vi "Chemical_Plant.vi"() -> ()   [LabVIEW 2024]
uses:
  <vilib>/addons/control/pid/pid.llb/PID (DBL).vi
  <vilib>/addons/control/pid/NI_PID_pid.lvlib
panel:
  in  "CHEMICAL PLANT":enum32{"MAIN_PANEL", "DSC", "FUNCTIONAL"}(tab)
  out "TRANS":bool
  in  "TRANSFORMER":bool
  out "Boolean 18":bool
  out "IL":dbl(knob) scale=0.0..200.0
  out "UL":dbl(knob) scale=0.0..10000.0
  out "TEMP 2":dbl(slide)=35.0 scale=0.0..1000.0
  in  "Power 2":i64(knob)=10 scale=0.0..10.0
  in  "Setpoint °C 2":dbl(knob)=1000.0 min=0.0 max=1000.0 step=1.0 scale=0.0..1000.0
  in  "CONV":bool
  out "Boolean 17":bool
  out "ATM":dbl(knob) scale=0.0..10.0
  out "Boolean 16":bool
  out "Boolean 15":bool
  in  "AV":bool
  in  "AP":bool
  out "Boolean 14":bool
  out "Boolean 13":bool
  in  "MV":bool
  in  "MP":bool
  out "Boolean 12":bool
  out "Boolean 11":bool
  in  "WV":bool
  in  "WP":bool
  out "Boolean 10":bool
  in  "CCV 2":bool
  out "Boolean 9":bool
  out "Boolean 8":bool
  in  "CCV":bool
  in  "CCP":bool
  in  "Set  limit":dbl=4.5 min=0.0 max=10.0 step=0.5 format="%#_2g"
  in  "COMP":bool
  out "Boolean 5":bool
  out "I_opv":dbl=0.9017177176073305
  out "U_opv":dbl=0.9017177176073305
  out "COMPRESSOR_ON":bool
  out "Boolean 7":bool
  in  "OPV":bool
  out "Boolean 6":bool
  in  "CV":bool
  in  "Slide Water":dbl(slide) scale=0.0..100.0
  in  "REFILL \nWATER TANK":bool
  out "TEMP":dbl(slide)=35.0 scale=0.0..1500.0
  in  "Power":i64(knob)=10 scale=0.0..10.0
  in  "Set  debit":dbl=0.25 min=0.0 max=1.0 step=0.05 format="%#_2g"
  out "Boolean 2":bool
  out "Boolean":bool
  in  "SV":bool
  in  "SP":bool
  in  "Slide Sulphur":dbl(slide) scale=0.0..100.0
  out "AIR QUALITY":dbl(knob) scale=0.0..10.0
  out "IL":dbl format="%#.2g"
  out "UL":dbl format="%#_5g"
  out "Res1":bool
  out "Thermometer\nConvertor":dbl(slide) scale=0.0..1000.0
  out "Thermometer\nFurnace":dbl(slide)=35.0 scale=0.0..1500.0
  out "I_f":dbl format="%#.2g"
  out "U_f":dbl format="%#.2g"
  out "I_av":dbl
  out "U_av":dbl
  out "I_ap":dbl
  out "U_ap":dbl
  out "I_wv":dbl
  out "U_wv":dbl
  out "I_wp":dbl
  out "U_wp":dbl
  out "I_mv":dbl
  out "U_mv":dbl
  out "I_mp":dbl
  out "U_mp":dbl
  out "I_ccv2":dbl
  out "U_ccv2":dbl
  out "I_cc":dbl
  out "U_cc":dbl
  out "I_ccp":dbl
  out "U_ccp":dbl
  out "I_ccv":dbl
  out "U_ccv":dbl
  out "I_c":dbl=0.3946202126362697
  out "U_c":dbl=0.3946202126362697
  out "I_cv":dbl format="%#.2g"
  out "U_cv":dbl format="%#.2g"
  out "I_sv":dbl format="%#.2g"
  out "U_sv":dbl format="%#.2g"
  out "I_sp":dbl=0.9017177176073305 format="%#.2g"
  out "U_sp":dbl=0.9017177176073305 format="%#.2g"
  out "PG_ONLINE":bool
  out "PP_ONLINE":bool
  out "TRANSFORMER_ON":bool
  out "HV_SWITCH_ON":bool
  out "PID1":bool
  out "PID2":bool
  out "PID3":bool
  out "CONVERTOR_ON":bool
  out "Acid2":bool
  out "Acid1":bool
  out "Acid Pump":bool
  out "Acid Valve":bool
  out "Water2":bool
  out "Abs2":bool
  out "Material Pump":bool
  out "Material Valve":bool
  out "Water Pump":bool
  out "Water Valve":bool
  out "Water1":bool
  out "Abs1":bool
  out "Catalyst3":bool
  out "Convertor Valve  2":bool
  out "ABSORTION TOWER":dbl(slide) scale=0.0..100.0
  out "WATER TANK":dbl(slide) scale=0.0..100.0
  out "FINAL PRODUCT\nTANK":dbl(slide) scale=0.0..100.0
  out "Catalityc Pump":bool
  out "DILUTION TOWER":dbl(slide) scale=0.0..100.0
  out "CATALYTIC \nCONVERTOR":dbl(slide) scale=0.0..100.0
  out "Pressure":dbl(knob)=1.0 scale=0.0..10.0
  out "Catalyst2":bool
  out "Catlytic Valve":bool
  out "Catalyst1":bool
  out "Pressure2":bool
  out "Pressure1":bool
  out "OverPressure\nValve":bool
  out "Comp 1":bool
  out "Compressor Valve":bool
  out "Comp 2":bool
  out "COMPRESSOR":dbl(slide) scale=0.0..100.0
  out "FURNACE_ON":bool
  out "FURNACE":dbl(slide) scale=0.0..100.0
  out "Sulphur Pump":bool
  out "Sulphur Valve":bool
  out "Sulf3":bool
  out "Sulf2":bool
  out "Sulf1":bool
  out "SULPHUR":dbl(slide) scale=0.0..100.0
  in  "stop":bool
  out "RESIDUAL WATER \nTANK":dbl(slide) scale=0.0..100.0
  in  "REFILL \nSULPHUR TANK":bool
  in  "Setpoint °C":dbl(knob)=1000.0 min=0.0 max=1500.0 step=1.0 scale=0.0..1500.0
  in  "PID gains":T1={"proportional gain (Kc)"=2.0, "integral time (Ti, min)"=0.05, "derivative time (Td, min)"=0.1} {"derivative time (Td, min)" format="%.3f"; "integral time (Ti, min)" format="%.3f"; "proportional gain (Kc)" format="%.3f"}
  out "output PID1":dbl format="%.2f"
  in  "FURN":bool
  out "Boolean 3":bool
  in  "HV_SW":bool
  out "Boolean 4":bool
  in  "Setpoint ATM":dbl(knob)=4.0 min=1.0 max=10.0 step=0.05 scale=1.0..10.0
  in  "PID gains 2":T1={"proportional gain (Kc)"=2.0, "integral time (Ti, min)"=0.05, "derivative time (Td, min)"=1.0} {"derivative time (Td, min)" format="%.3f"; "integral time (Ti, min)" format="%.3f"; "proportional gain (Kc)" format="%.3f"}
  out "output PID2":dbl format="%.2f"
  out "output PID3":dbl format="%.2f"
  in  "PID gains 3":T1={"proportional gain (Kc)"=2.0, "integral time (Ti, min)"=0.05, "derivative time (Td, min)"=0.1} {"derivative time (Td, min)" format="%.3f"; "integral time (Ti, min)" format="%.3f"; "proportional gain (Kc)" format="%.3f"}
  # "CONTROLS"
  # "CHEMICAL PROCESS"
  # "BUJOAIA \nCHEMICAL COMPLEX"
  # "FLOW CONTROL"
  # "AUTO*\ndefault\nopen on \nlimit ser"
  # "FURNACE"
  # "COMPRESSOR"
  # "CONVERTOR"
  # "ELECTRICAL SYSTEM"
  # "ELECTRICAL SYSTEM"
  # "110kV Power Substation"
  # "110kV Power Grid"
  # "POWER PLANT"
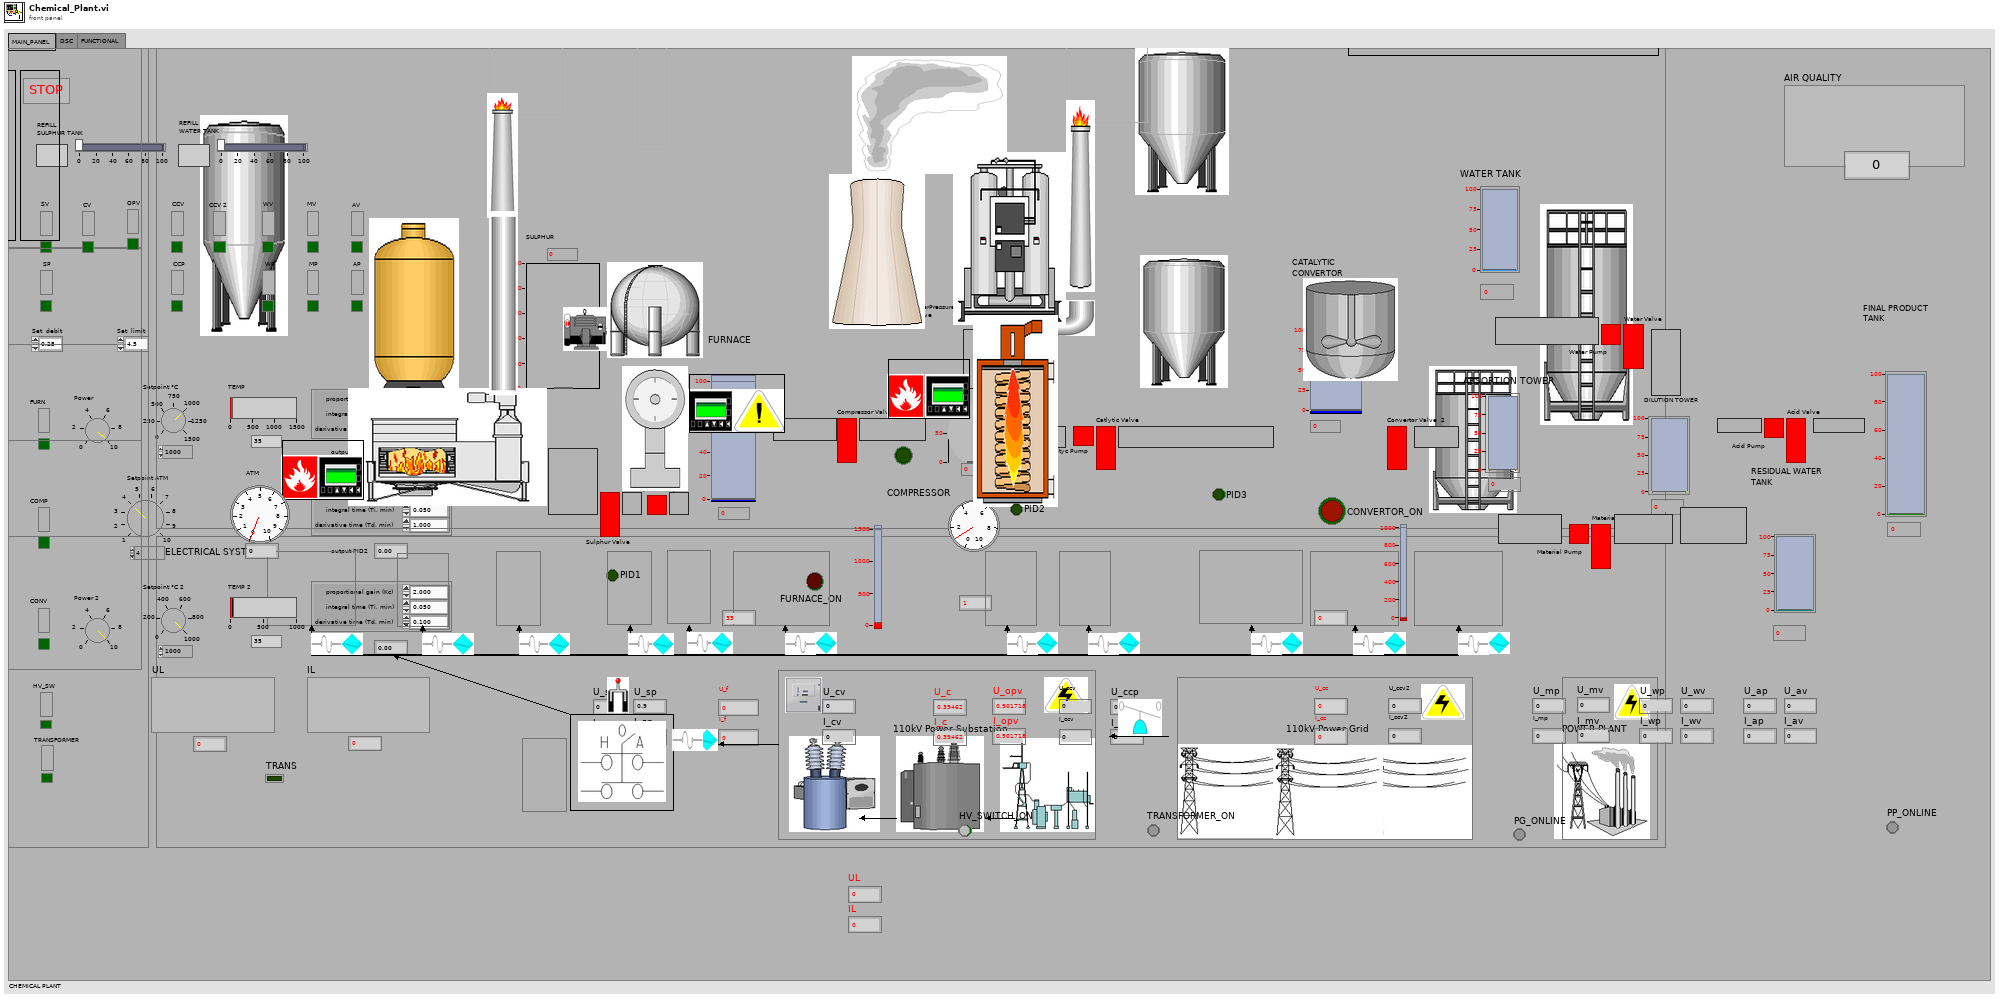
[diagram p1: front panel]
types:
  T1 = cluster{"proportional gain (Kc)":dbl, "integral time (Ti, min)":dbl, "derivative time (Td, min)":dbl}
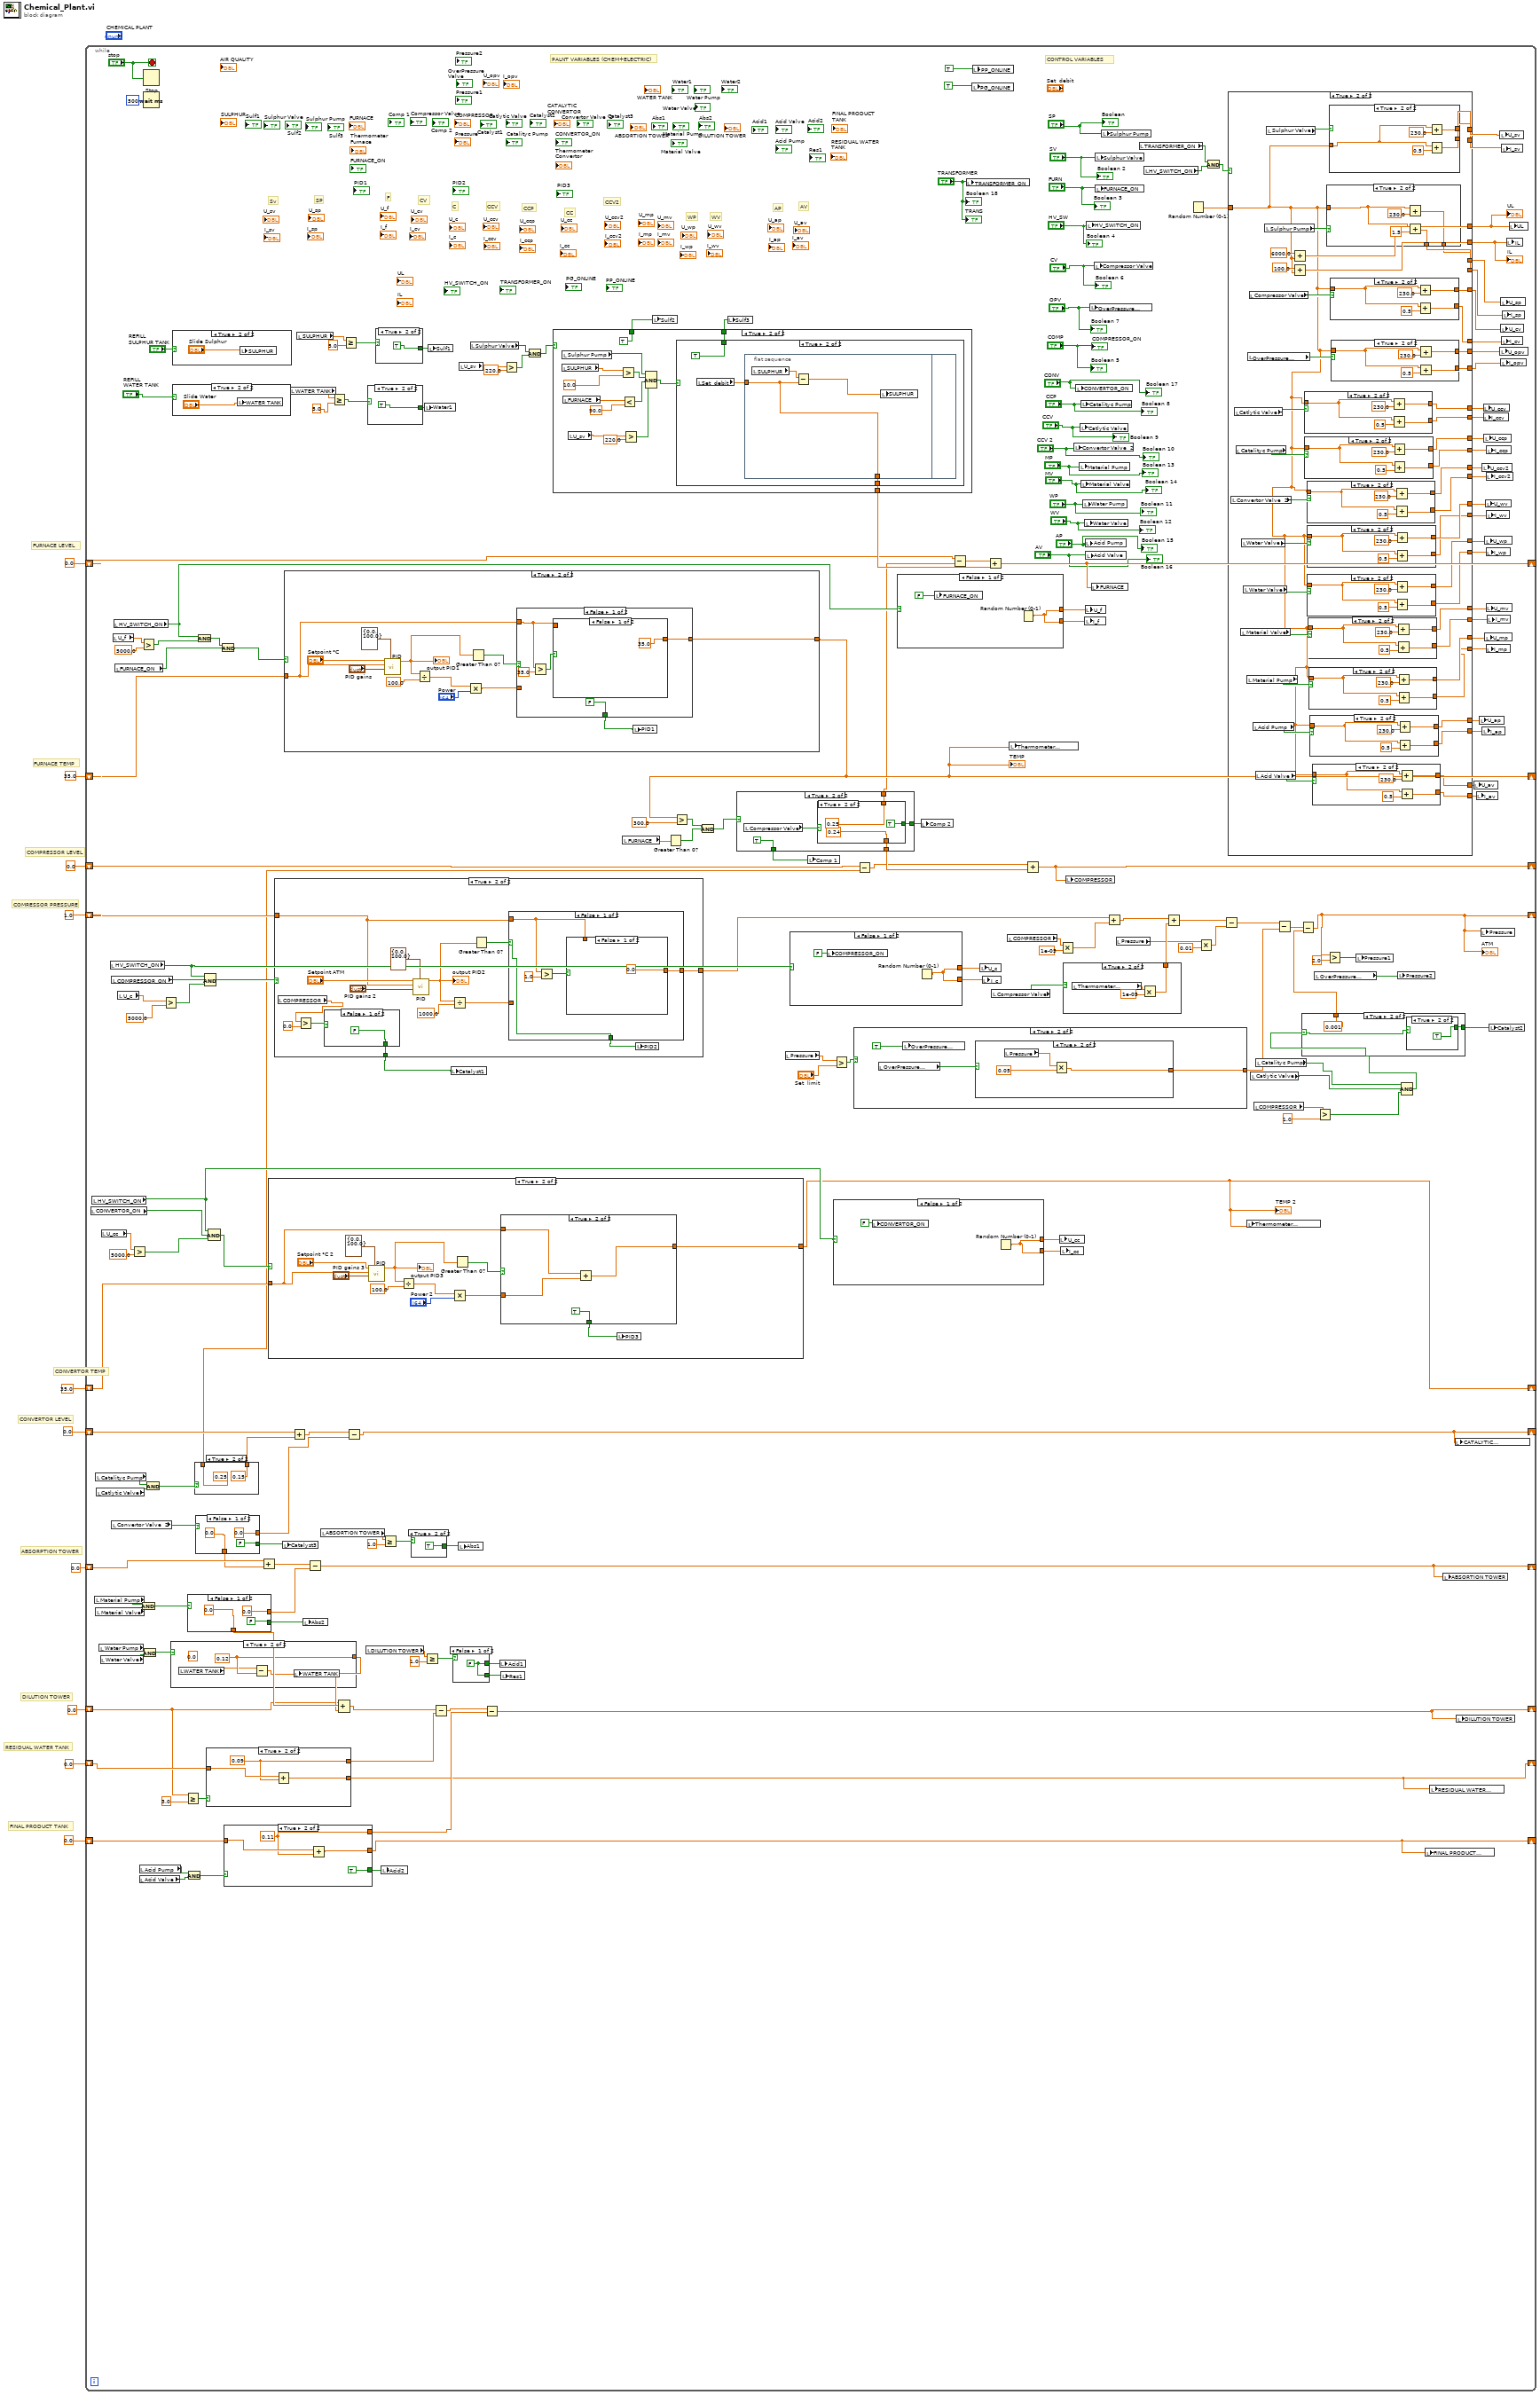
[diagram p0: block diagram]
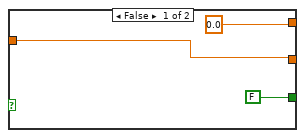
[diagram p2: hidden frame]
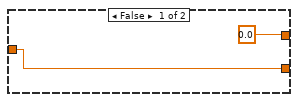
[diagram p3: hidden frame]
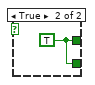
[diagram p4: hidden frame]
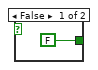
[diagram p5: hidden frame]
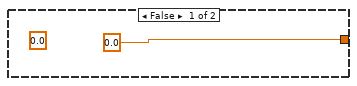
[diagram p6: hidden frame]
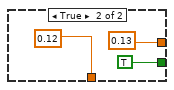
[diagram p7: hidden frame]
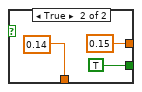
[diagram p8: hidden frame]
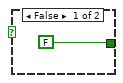
[diagram p9: hidden frame]
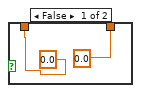
[diagram p11: hidden frame]
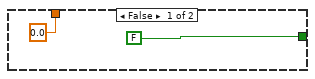
[diagram p12: hidden frame]
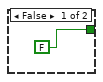
[diagram p13: hidden frame]
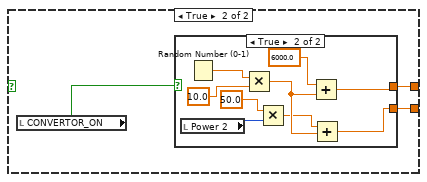
[diagram p14: hidden frame]
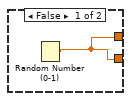
[diagram p15: hidden frame]
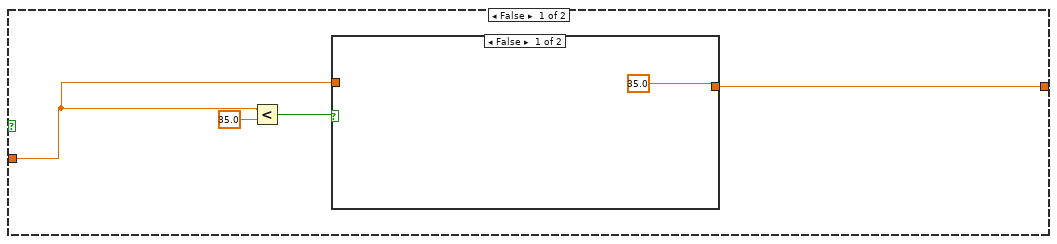
[diagram p16: hidden frame]
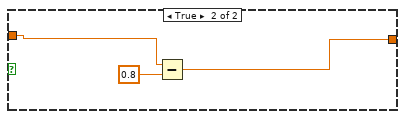
[diagram p17: hidden frame]
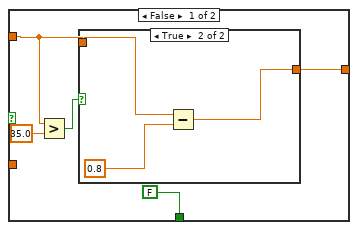
[diagram p18: hidden frame]
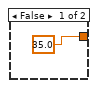
[diagram p19: hidden frame]
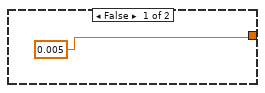
[diagram p20: hidden frame]
diagram:
  # "FINAL PRODUCT TANK"
  # "RESIDUAL WATER TANK"
  # "DILUTION TOWER"
  # "ABSORPTION TOWER"
  # "CONVERTOR LEVEL"
  # "CONVERTOR TEMP"
  # "COMRESSOR PRESSURE"
  # "COMPRESSOR LEVEL"
  # "FURNACE TEMP"
  # "FURNACE LEVEL"
  n1 = while {
    shift-right: [w196] -> _
    shift-left: 0.0 -> [w180]
    shift-right: [w183] -> _
    shift-left: 35.0 -> [w189]
    shift-right: [w177] -> _
    shift-left: 0.0 -> [w69]
    shift-right: [w84] -> _
    shift-left: 1.0 -> [w152]
    shift-right: [w86] -> _
    shift-left: 35.0 -> [w95]
    shift-right: [w66] -> _
    shift-left: 0.0 -> [w71]
    shift-right: [w55] -> _
    shift-left: 0.0 -> [w57]
    shift-right: [w31] -> _
    shift-left: 0.0 -> [w29]
    shift-right: [w19] -> _
    shift-left: 0.0 -> [w35]
    shift-right: [w20] -> _
    shift-left: 0.0 -> [w24]
    stop <- "stop" stop-if-true
    # "CONTROL VARIABLES"
    # "PALNT VARIABLES (CHEM+ELECTRIC)"
    # "C"
    # "WV"
    # "WP"
    # "CV"
    # "AV"
    # "AP"
    # "CC"
    # "CCV2"
    # "CCP"
    # "CCV"
    # "F"
    # "SP"
    # "Sv"
    n2 = local read "CONVERTOR_ON"() -> (w88:bool)
    n3 = local read "HV_SWITCH_ON"() -> (w87:bool)
    n4 = local read "Material Pump"() -> (w52:bool)
    n5 = local read "Catalityc Pump"() -> (w75:bool)
    n6 = local read "Material Valve"() -> (w51:bool)
    n7 = local read "Catlytic Valve"() -> (w74:bool)
    n8 = local read "Water Pump"() -> (w50:bool)
    n9 = local read "Water Valve"() -> (w49:bool)
    n10 = local read "U_cc"() -> (w89:dbl)
    n11 = local read "HV_SWITCH_ON"() -> (w146:bool)
    n12 = local read "COMPRESSOR_ON"() -> (w150:bool)
    n13 = local read "Convertor Valve  2"() -> (w60:bool)
    n14 = local read "U_f"() -> (w195:dbl)
    n15 = local read "HV_SWITCH_ON"() -> (w186:bool)
    n16 = local read "FURNACE_ON"() -> (w191:bool)
    n17 = local read "U_c"() -> (w147:dbl)
    n18 = Greater?(x=w89, y=5000.0) -> (0:w91:bool)
    n19 = local read "Acid Pump"() -> (w26:bool)
    n20 = local read "Acid Valve"() -> (w25:bool)
    n21 = And(x=w52, y=w51) -> (x .and. y?=w54:bool)
    n22 = Greater?(x=w195, y=5000.0) -> (0:w193:bool)
    n23 = And(x=w50, y=w49) -> (x .and. y?=w53:bool)
    n24 = Stop(stop? (T)="stop") -> ()
    n25 = Wait (ms)(milliseconds to wait=u32 500) -> ()  [unwired: 1 out]
    n26 = And(x=w75, y=w74) -> (x .and. y?=w73:bool)
    n27 = Greater?(x=w147, y=5000.0) -> (0:w149:bool)
    n28 = case shown="True" w53 {
      tunnel: [0.0 w226] -> w45
      frame False {
        (unwired) 0.0
      }
      frame True {
        w226 = 0.12
        (unwired) 0.0
        n29 = local read "WATER TANK"() -> (w225:dbl)
        n30 = Subtract(x=w225, y=w226) -> (x-y=w227:dbl)
        n31 = local write "WATER TANK"(w227) -> ()
      }
    }
    n32 = case shown="True" "REFILL \nWATER TANK" {
      frame False {
      }
      frame True {
        n33 = local write "WATER TANK"("Slide Water") -> ()
      }
    }
    n34 = case shown="True" "REFILL \nSULPHUR TANK" {
      frame False {
      }
      frame True {
        n35 = local write "SULPHUR"("Slide Sulphur") -> ()
      }
    }
    n36 = Greater Or Equal?(x=w29, y=3.0) -> (x >= y?=w28:bool)
    n37 = And(x=w26, y=w25) -> (x .and. y?=w27:bool)
    n38 = case shown="False" w54 {
      tunnel: [0.0 0.13] -> w48
      tunnel: [0.0 0.12] -> w47
      tunnel: [FALSE TRUE] -> w21
      frame False {
      }
      frame True {
      }
    }
    n39 = case shown="True" w73 {
      tunnel: [0.0 0.15] -> w72
      tunnel: [0.0 0.25] -> w68
      frame False {
      }
      frame True {
      }
    }
    n40 = case shown="False" w60 {
      tunnel: [0.0 0.15] -> w59
      tunnel: [0.0 0.14] -> w56
      tunnel: [FALSE TRUE] -> w46
      frame False {
      }
      frame True {
      }
    }
    n41 = And(x=w186, y=w193) -> (x .and. y?=w192:bool)
    n42 = Compound Arithmetic op=AND(w146, w150, w149) -> (w151:bool)
    n43 = case shown="True" w28 {
      tunnel: w35 -> [w215 w219]
      tunnel: [w215 w218] -> w19
      tunnel: [0.0 w217] -> w33
      frame False {
      }
      frame True {
        w217 = 0.09
        n44 = Add(x=w219, y=w217) -> (x+y=w218:dbl)
      }
    }
    n45 = Compound Arithmetic op=AND(w87, w88, w91) -> (w92:bool)
    n46 = And(x=w192, y=w191) -> (x .and. y?=w190:bool)
    n47 = case shown="True" w27 {
      tunnel: w24 -> [w209 w214]
      tunnel: [0.0 w213] -> w23
      tunnel: [w209 w212] -> w20
      tunnel: [FALSE TRUE] -> w22
      frame False {
      }
      frame True {
        w213 = 0.11
        n48 = Add(x=w214, y=w213) -> (x+y=w212:dbl)
      }
    }
    n49 = Add(x=w57, y=w56) -> (x+y=w58:dbl)
    n50 = case shown="True" w92 {
      tunnel: w95 -> [w270 w285]
      tunnel: [w269 w284] -> w86
      frame False {
        n51 = Less?(x=w270, y=35.0) -> (x < y?=w272:bool)
        n52 = case shown="False" w272 {
          tunnel: w270 -> [_ w275]
          tunnel: [35.0 w274] -> w269
          frame False {
          }
          frame True {
            n53 = Subtract(x=w275, y=0.8) -> (x-y=w274:dbl)
          }
        }
      }
      frame True {
        n54 = call-poly <vilib>:"PID.vi"("output range"=cluster{"output high":dbl, "output low":dbl} {"output high"=0.0, "output low"=100.0}, "PID gains"="PID gains 3", "process variable"=w285, "setpoint"="Setpoint °C 2") -> ("output"=w280:dbl)  [unwired: 6 in, 1 out]
        "output PID3" <- w280
        n55 = Divide(x=w280, y=100.0) -> (x/y=w282:dbl)
        n56 = Multiply(x=w282, y="Power 2") -> (x*y=w283:dbl)
        n57 = Greater Than 0?(x=w280) -> (x > 0?=w281:bool)
        n58 = case shown="True" w281 {
          tunnel: w285 -> [w290 w301]
          tunnel: [w293 w300] -> w284
          tunnel: w283 -> [_ w299]
          tunnel: [FALSE TRUE] -> w279
          frame False {
            n59 = Greater?(x=w290, y=35.0) -> (0:w291:bool)
            n60 = case shown="True" w291 {
              tunnel: w290 -> [_ w296]
              tunnel: [35.0 w295] -> w293
              frame False {
              }
              frame True {
                n61 = Subtract(x=w296, y=0.8) -> (x-y=w295:dbl)
              }
            }
          }
          frame True {
            n62 = Add(x=w301, y=w299) -> (x+y=w300:dbl)
          }
        }
        n63 = local write "PID3"(w279) -> ()
      }
    }
    "TEMP 2" <- w86
    n64 = case shown="True" w151 {
      tunnel: w152 -> [w331 w342]
      tunnel: [w330 w344] -> w141
      tunnel: [FALSE w341] -> w127
      frame False {
        n65 = Greater?(x=w331, y=1.0) -> (0:w333:bool)
        n66 = case shown="False" w333 {
          tunnel: w331 -> [_ w336]
          tunnel: [1.0 w335] -> w330
          frame False {
          }
          frame True {
            n67 = Subtract(x=w336, y=0.05) -> (x-y=w335:dbl)
          }
        }
      }
      frame True {
        n68 = local read "COMPRESSOR"() -> (w338:dbl)
        n69 = Greater?(x=w338, y=0.0) -> (0:w340:bool)
        n70 = case shown="False" w340 {
          tunnel: [FALSE TRUE] -> w341
          frame False {
          }
          frame True {
          }
        }
        n71 = call-poly <vilib>:"PID.vi"("output range"=cluster{"output high":dbl, "output low":dbl} {"output high"=0.0, "output low"=100.0}, "PID gains"="PID gains 2", "process variable"=w342, "setpoint"="Setpoint ATM") -> ("output"=w345:dbl)  [unwired: 6 in, 1 out]
        "output PID2" <- w345
        n72 = Divide(x=w345, y=1000.0) -> (x/y=w347:dbl)
        n73 = Greater Than 0?(x=w345) -> (x > 0?=w346:bool)
        n74 = case shown="False" w346 {
          selector: w346 -> [w357 w366]
          tunnel: w347 -> [_ w364]
          tunnel: [w358 w365] -> w344
          tunnel: [w357 w366] -> w343
          tunnel: w342 -> [w354 w363]
          frame False {
            n75 = Greater?(x=w354, y=1.0) -> (0:w356:bool)
            n76 = case shown="False" w356 {
              tunnel: [0.0 w361] -> w358
              tunnel: w354 -> [_ w360]
              frame False {
              }
              frame True {
                n77 = Subtract(x=w360, y=0.05) -> (x-y=w361:dbl)
              }
            }
          }
          frame True {
            n78 = Add(x=w363, y=w364) -> (x+y=w365:dbl)
          }
        }
        n79 = local write "PID2"(w343) -> ()
      }
    }
    n80 = local write "Catalyst3"(w46) -> ()
    n81 = case shown="True" w190 {
      tunnel: w189 -> [w521 w534]
      tunnel: [w520 w533] -> w183
      frame False {
        n82 = Less?(x=w521, y=35.0) -> (x < y?=w523:bool)
        n83 = case shown="False" w523 {
          tunnel: w521 -> [_ w526]
          tunnel: [35.0 w525] -> w520
          frame False {
          }
          frame True {
            n84 = Subtract(x=w526, y=0.8) -> (x-y=w525:dbl)
          }
        }
      }
      frame True {
        n85 = call-poly <vilib>:"PID.vi"("output range"=cluster{"output high":dbl, "output low":dbl} {"output high"=0.0, "output low"=100.0}, "PID gains"="PID gains", "process variable"=w534, "setpoint"="Setpoint °C") -> ("output"=w529:dbl)  [unwired: 6 in, 1 out]
        "output PID1" <- w529
        n86 = Divide(x=w529, y=100.0) -> (x/y=w531:dbl)
        n87 = Multiply(x=w531, y="Power") -> (x*y=w532:dbl)
        n88 = Greater Than 0?(x=w529) -> (x > 0?=w530:bool)
        n89 = case shown="False" w530 {
          tunnel: w534 -> [w541 w552]
          tunnel: [w544 w551] -> w533
          tunnel: w532 -> [_ w550]
          tunnel: [FALSE TRUE] -> w528
          frame False {
            n90 = Greater?(x=w541, y=35.0) -> (0:w542:bool)
            n91 = case shown="False" w542 {
              tunnel: w541 -> [_ w547]
              tunnel: [35.0 w546] -> w544
              frame False {
              }
              frame True {
                n92 = Subtract(x=w547, y=0.8) -> (x-y=w546:dbl)
              }
            }
          }
          frame True {
            n93 = Add(x=w552, y=w550) -> (x+y=w551:dbl)
          }
        }
        n94 = local write "PID1"(w528) -> ()
      }
    }
    "TEMP" <- w183
    n95 = local read "WATER TANK"() -> (w64:dbl)
    n96 = Add(x=w71, y=w72) -> (x+y=w67:dbl)
    n97 = local read "SULPHUR"() -> (w206:dbl)
    n98 = local write "Abs2"(w21) -> ()
    n99 = Subtract(x=w58, y=w48) -> (x-y=w55:dbl)
    n100 = local read "ABSORTION TOWER"() -> (w41:dbl)
    n101 = Greater Or Equal?(x=w64, y=5.0) -> (x >= y?=w62:bool)
    n102 = Compound Arithmetic op=ADD(w29, w47, w45) -> (w34:dbl)
    n103 = Greater Or Equal?(x=w206, y=5.0) -> (x >= y?=w204:bool)
    n104 = Subtract(x=w67, y=w59) -> (x-y=w66:dbl)
    n105 = local read "DILUTION TOWER"() -> (w37:dbl)
    n106 = case shown="True" w62 {
      tunnel: [FALSE TRUE] -> w61
      frame False {
      }
      frame True {
      }
    }
    n107 = case shown="True" w204 {
      tunnel: [FALSE TRUE] -> w203
      frame False {
      }
      frame True {
      }
    }
    n108 = local write "Acid2"(w22) -> ()
    n109 = Greater Or Equal?(x=w41, y=1.0) -> (x >= y?=w43:bool)
    n110 = case shown="True" w43 {
      tunnel: [FALSE TRUE] -> w44
      frame False {
      }
      frame True {
      }
    }
    n111 = local write "Water1"(w61) -> ()
    n112 = Greater Or Equal?(x=w37, y=1.0) -> (x >= y?=w39:bool)
    n113 = local write "Sulf1"(w203) -> ()
    n114 = Subtract(x=w34, y=w33) -> (x-y=w32:dbl)
    n115 = local write "Catalyst1"(w127) -> ()
    n116 = case shown="False" w39 {
      tunnel: [w220 w221] -> w40
      tunnel: [w220 w221] -> w36
      frame False {
        w220 = FALSE
      }
      frame True {
        w221 = TRUE
      }
    }
    n117 = local write "Abs1"(w44) -> ()
    n118 = local read "U_sv"() -> (w160:dbl)
    n119 = local read "Sulphur Valve"() -> (w163:bool)
    n120 = Subtract(x=w32, y=w23) -> (x-y=w31:dbl)
    n121 = local write "Acid1"(w40) -> ()
    n122 = local write "Res1"(w36) -> ()
    n123 = Greater?(x=w160, y=220.0) -> (0:w161:bool)
    n124 = And(x=w163, y=w161) -> (x .and. y?=w162:bool)
    n125 = case shown="True" w162 {
      tunnel: [FALSE TRUE] -> w201
      tunnel: [FALSE w568] -> w197
      tunnel: [0.0 w563] -> w185
      frame False {
      }
      frame True {
        n126 = local read "SULPHUR"() -> (w564:dbl)
        n127 = local read "Sulphur Pump"() -> (w561:bool)
        n128 = local read "FURNACE"() -> (w566:dbl)
        n129 = local read "U_sv"() -> (w556:dbl)
        n130 = Greater?(x=w564, y=10.0) -> (0:w560:bool)
        n131 = Less?(x=w566, y=90.0) -> (x < y?=w559:bool)
        n132 = Greater?(x=w556, y=220.0) -> (0:w557:bool)
        n133 = Compound Arithmetic op=AND(w561, w560, w559, w557) -> (w562:bool)
        n134 = case shown="True" w562 {
          tunnel: [FALSE TRUE] -> w568
          tunnel: [0.0 w573] -> w563
          frame False {
            n135 = local write "Sulphur Pump"(FALSE) -> ()
          }
          frame True {
            n136 = local read "Set  debit"() -> (w574:dbl)
            n137 = flat-sequence {
              tunnel: w574 -> [w576]
              tunnel: [w576] -> w573
              frame #0 {
                n138 = local read "SULPHUR"() -> (w578:dbl)
                n139 = Subtract(x=w578, y=w576) -> (x-y=w577:dbl)
                n140 = local write "SULPHUR"(w577) -> ()
              }
              frame #1 {
              }
            }
          }
        }
      }
    }
    n141 = local read "FURNACE"() -> (w174:dbl)
    n142 = local write "Sulf2"(w201) -> ()
    n143 = Greater Than 0?(x=w174) -> (x > 0?=w173:bool)
    n144 = Greater?(x=w183, y=300.0) -> (0:w176:bool)
    n145 = And(x=w176, y=w173) -> (x .and. y?=w175:bool)
    n146 = local write "Sulf3"(w197) -> ()
    n147 = case shown="True" w175 {
      tunnel: [w493 w497] -> w179
      tunnel: [w493 w496] -> w178
      tunnel: [FALSE TRUE] -> w172
      tunnel: [FALSE w494] -> w171
      frame False {
        w493 = 0.0
      }
      frame True {
        n148 = local read "Compressor Valve"() -> (w498:bool)
        n149 = case shown="True" w498 {
          tunnel: [0.005 0.25] -> w497
          tunnel: [0.0 0.24] -> w496
          tunnel: [FALSE TRUE] -> w494
          frame False {
          }
          frame True {
          }
        }
      }
    }
    n150 = local read "Pressure"() -> (w129:dbl)
    n151 = case shown="False" w146 {
      tunnel: [w314 w318] -> w139
      tunnel: [w314 w317] -> w138
      frame False {
        n152 = local write "COMPRESSOR_ON"(FALSE) -> ()
        n153 = Random Number (0-1)() -> (number: 0 to 1=w314:dbl)
      }
      frame True {
        n154 = local read "COMPRESSOR_ON"() -> (w316:bool)
        n155 = case shown="True" w316 {
          tunnel: [w319 w324] -> w318
          tunnel: [w319 w323] -> w317
          frame False {
            n156 = Random Number (0-1)() -> (number: 0 to 1=w319:dbl)
          }
          frame True {
            n157 = local read "Setpoint ATM"() -> (w320:dbl)
            n158 = Random Number (0-1)() -> (number: 0 to 1=w327:dbl)
            n159 = Multiply(x=w327, y=10.0) -> (x*y=w328:dbl)
            n160 = Multiply(x=50.0, y=w320) -> (x*y=w322:dbl)
            n161 = Add(x=6000.0, y=w328) -> (x+y=w324:dbl)
            n162 = Add(x=w322, y=w328) -> (x+y=w323:dbl)
          }
        }
      }
    }
    n163 = local write "Comp 1"(w172) -> ()
    n164 = case shown="False" w87 {
      tunnel: [w255 w257] -> w94
      tunnel: [w255 w256] -> w93
      frame False {
        n165 = local write "CONVERTOR_ON"(FALSE) -> ()
        n166 = Random Number (0-1)() -> (number: 0 to 1=w255:dbl)
      }
      frame True {
        n167 = local read "CONVERTOR_ON"() -> (w258:bool)
        n168 = case shown="True" w258 {
          tunnel: [w259 w264] -> w257
          tunnel: [w259 w263] -> w256
          frame False {
            n169 = Random Number (0-1)() -> (number: 0 to 1=w259:dbl)
          }
          frame True {
            n170 = local read "Power 2"() -> (w260:i64)
            n171 = Random Number (0-1)() -> (number: 0 to 1=w267:dbl)
            n172 = Multiply(x=w267, y=10.0) -> (x*y=w268:dbl)
            n173 = Multiply(x=50.0, y=w260) -> (x*y=w262:dbl)
            n174 = Add(x=6000.0, y=w268) -> (x+y=w264:dbl)
            n175 = Add(x=w262, y=w268) -> (x+y=w263:dbl)
          }
        }
      }
    }
    n176 = Greater?(x=w129, y="Set  limit") -> (0:w131:bool)
    n177 = case shown="True" w131 {
      tunnel: [0.005 w303] -> w130
      frame False {
      }
      frame True {
        n178 = local read "OverPressure\nValve"() -> (w304:bool)
        n179 = local write "OverPressure\nValve"(TRUE) -> ()
        n180 = case shown="True" w304 {
          tunnel: [0.001 w307] -> w303
          frame False {
          }
          frame True {
            n181 = local read "Pressure"() -> (w309:dbl)
            n182 = Multiply(x=w309, y=0.05) -> (x*y=w307:dbl)
          }
        }
      }
    }
    n183 = Subtract(x=w69, y=w68) -> (x-y=w70:dbl)
    n184 = case shown="False" w186 {
      tunnel: [w505 w509] -> w170
      tunnel: [w505 w508] -> w169
      frame False {
        n185 = local write "FURNACE_ON"(FALSE) -> ()
        n186 = Random Number (0-1)() -> (number: 0 to 1=w505:dbl)
      }
      frame True {
        n187 = local read "FURNACE_ON"() -> (w507:bool)
        n188 = case shown="True" w507 {
          tunnel: [w510 w515] -> w509
          tunnel: [w510 w514] -> w508
          frame False {
            n189 = Random Number (0-1)() -> (number: 0 to 1=w510:dbl)
          }
          frame True {
            n190 = local read "Power"() -> (w511:i64)
            n191 = Random Number (0-1)() -> (number: 0 to 1=w518:dbl)
            n192 = Multiply(x=w518, y=10.0) -> (x*y=w519:dbl)
            n193 = Multiply(x=50.0, y=w511) -> (x*y=w513:dbl)
            n194 = Add(x=6000.0, y=w519) -> (x+y=w515:dbl)
            n195 = Add(x=w513, y=w519) -> (x+y=w514:dbl)
          }
        }
      }
    }
    n196 = local write "Comp 2"(w171) -> ()
    n197 = Subtract(x=w180, y=w179) -> (x-y=w181:dbl)
    n198 = local write "TRANSFORMER_ON"("TRANSFORMER") -> ()
    n199 = local write "PG_ONLINE"(TRUE) -> ()
    n200 = local write "PP_ONLINE"(TRUE) -> ()
    n201 = local write "U_c"(w139) -> ()
    n202 = local write "I_c"(w138) -> ()
    n203 = Add(x=w181, y=w185) -> (x+y=w196:dbl)
    n204 = local read "Compressor Valve"() -> (w137:bool)
    n205 = local read "COMPRESSOR"() -> (w144:dbl)
    n206 = local write "Thermometer\nFurnace"(w183) -> ()
    n207 = Add(x=w70, y=w178) -> (x+y=w177:dbl)
    n208 = local write "U_cc"(w94) -> ()
    n209 = Multiply(x=w144, y=1e-05) -> (x*y=w143:dbl)
    n210 = local write "I_cc"(w93) -> ()
    n211 = case shown="True" w137 {
      tunnel: [0.0 w311] -> w142
      frame False {
      }
      frame True {
        n212 = local read "Thermometer\nFurnace"() -> (w312:dbl)
        n213 = Multiply(x=w312, y=1e-05) -> (x*y=w311:dbl)
      }
    }
    n214 = local write "COMPRESSOR"(w177) -> ()
    n215 = local write "Convertor Valve  2"("CCV 2") -> ()
    n216 = local write "CONVERTOR_ON"("CONV") -> ()
    n217 = local write "Material Pump"("MP") -> ()
    n218 = local write "Catlytic Valve"("CCV") -> ()
    n219 = local write "Catalityc Pump"("CCP") -> ()
    n220 = local write "Material Valve"("MV") -> ()
    n221 = local write "Water Pump"("WP") -> ()
    n222 = local write "Water Valve"("WV") -> ()
    n223 = local write "I_f"(w169) -> ()
    n224 = local write "Acid Pump"("AP") -> ()
    n225 = local write "U_f"(w170) -> ()
    n226 = local write "Acid Valve"("AV") -> ()
    n227 = local write "HV_SWITCH_ON"("HV_SW") -> ()
    n228 = local write "OverPressure\nValve"("OPV") -> ()
    n229 = local write "FURNACE"(w196) -> ()
    n230 = local write "Compressor Valve"("CV") -> ()
    n231 = local write "Sulphur Valve"("SV") -> ()
    n232 = local write "FURNACE_ON"("FURN") -> ()
    n233 = local write "Sulphur Pump"("SP") -> ()
    n234 = Add(x=w141, y=w143) -> (x+y=w140:dbl)
    n235 = local read "Pressure"() -> (w134:dbl)
    n236 = local read "TRANSFORMER_ON"() -> (w16:bool)
    n237 = local read "HV_SWITCH_ON"() -> (w18:bool)
    n238 = Add(x=w140, y=w142) -> (x+y=w136:dbl)
    n239 = Random Number (0-1)() -> (number: 0 to 1=w168:dbl)
    n240 = Multiply(x=w134, y=0.01) -> (x*y=w135:dbl)
    n241 = And(x=w16, y=w18) -> (x .and. y?=w17:bool)
    n242 = Subtract(x=w136, y=w135) -> (x-y=w132:dbl)
    n243 = case shown="True" w17 {
      tunnel: w168 -> [w368 w373]
      tunnel: [w368 w410] -> w167
      tunnel: [w368 w409] -> w166
      tunnel: [w368 w408] -> w165
      tunnel: [w368 w407] -> w164
      tunnel: [w368 w403] -> w14
      tunnel: [w368 w404] -> w13
      tunnel: [w368 w401] -> w158
      tunnel: [w368 w399] -> w157
      tunnel: [w368 w398] -> w156
      tunnel: [w368 w397] -> w155
      tunnel: [w368 w386] -> w123
      tunnel: [w368 w385] -> w122
      tunnel: [w368 w384] -> w121
      tunnel: [w368 w383] -> w120
      tunnel: [w368 w387] -> w119
      tunnel: [w368 w388] -> w118
      tunnel: [w368 w389] -> w117
      tunnel: [w368 w390] -> w116
      tunnel: [w368 w391] -> w115
      tunnel: [w368 w392] -> w114
      tunnel: [w368 w393] -> w113
      tunnel: [w368 w394] -> w112
      tunnel: [w368 w395] -> w111
      tunnel: [w368 w396] -> w110
      tunnel: [w368 w372] -> w100
      tunnel: [w368 w371] -> w99
      tunnel: [w368 w370] -> w98
      tunnel: [w368 w369] -> w97
      frame False {
        w367 = FALSE
        n244 = local write "OverPressure\nValve"(w367) -> ()
        n245 = local write "Catlytic Valve"(w367) -> ()
        n246 = local write "Catalityc Pump"(w367) -> ()
        n247 = local write "Acid Pump"(w367) -> ()
        n248 = local write "Acid Valve"(w367) -> ()
        n249 = local write "Water Valve"(w367) -> ()
        n250 = local write "Material Valve"(w367) -> ()
        n251 = local write "Sulphur Pump"(w367) -> ()
        n252 = local write "Material Pump"(w367) -> ()
        n253 = local write "Water Pump"(w367) -> ()
        n254 = local write "Sulphur Valve"(w367) -> ()
        n255 = local write "Convertor Valve  2"(w367) -> ()
        n256 = local write "Compressor Valve"(w367) -> ()
      }
      frame True {
        n257 = local read "Convertor Valve  2"() -> (w380:bool)
        n258 = local read "Catlytic Valve"() -> (w382:bool)
        n259 = local read "Catalityc Pump"() -> (w381:bool)
        n260 = local read "Material Valve"() -> (w377:bool)
        n261 = local read "Water Valve"() -> (w379:bool)
        n262 = local read "Water Valve"() -> (w378:bool)
        n263 = local read "Material Pump"() -> (w376:bool)
        n264 = local read "OverPressure\nValve"() -> (w400:bool)
        n265 = local read "Compressor Valve"() -> (w402:bool)
        n266 = local read "Acid Pump"() -> (w375:bool)
        n267 = local read "Acid Valve"() -> (w374:bool)
        n268 = local read "Sulphur Pump"() -> (w411:bool)
        n269 = local read "Sulphur Valve"() -> (w412:bool)
        n270 = Add(x=6000.0, y=w373) -> (x+y=w404:dbl)
        n271 = Add(x=100.0, y=w373) -> (x+y=w403:dbl)
        n272 = case shown="True" w382 {
          tunnel: [w461 w464] -> w396
          tunnel: [w461 w463] -> w395
          tunnel: w373 -> [w461 w462]
          frame False {
          }
          frame True {
            n273 = Add(x=w462, y=230.0) -> (x+y=w464:dbl)
            n274 = Add(x=w462, y=0.5) -> (x+y=w463:dbl)
          }
        }
        n275 = case shown="True" w381 {
          tunnel: [w455 w458] -> w394
          tunnel: [w455 w457] -> w393
          tunnel: w373 -> [w455 w456]
          frame False {
          }
          frame True {
            n276 = Add(x=w456, y=230.0) -> (x+y=w458:dbl)
            n277 = Add(x=w456, y=0.5) -> (x+y=w457:dbl)
          }
        }
        n278 = case shown="True" w380 {
          tunnel: [w449 w452] -> w392
          tunnel: [w449 w451] -> w391
          tunnel: w373 -> [w449 w450]
          frame False {
          }
          frame True {
            n279 = Add(x=w450, y=230.0) -> (x+y=w452:dbl)
            n280 = Add(x=w450, y=0.5) -> (x+y=w451:dbl)
          }
        }
        n281 = case shown="True" w379 {
          tunnel: [w443 w446] -> w390
          tunnel: [w443 w445] -> w389
          tunnel: w373 -> [w443 w444]
          frame False {
          }
          frame True {
            n282 = Add(x=w444, y=230.0) -> (x+y=w446:dbl)
            n283 = Add(x=w444, y=0.5) -> (x+y=w445:dbl)
          }
        }
        n284 = case shown="True" w378 {
          tunnel: [w437 w440] -> w388
          tunnel: [w437 w439] -> w387
          tunnel: w373 -> [w437 w438]
          frame False {
          }
          frame True {
            n285 = Add(x=w438, y=230.0) -> (x+y=w440:dbl)
            n286 = Add(x=w438, y=0.5) -> (x+y=w439:dbl)
          }
        }
        n287 = case shown="True" w377 {
          tunnel: [w431 w434] -> w386
          tunnel: [w431 w433] -> w385
          tunnel: w373 -> [w431 w432]
          frame False {
          }
          frame True {
            n288 = Add(x=w432, y=230.0) -> (x+y=w434:dbl)
            n289 = Add(x=w432, y=0.5) -> (x+y=w433:dbl)
          }
        }
        n290 = case shown="True" w376 {
          tunnel: [w425 w428] -> w384
          tunnel: [w425 w427] -> w383
          tunnel: w373 -> [w425 w426]
          frame False {
          }
          frame True {
            n291 = Add(x=w426, y=230.0) -> (x+y=w428:dbl)
            n292 = Add(x=w426, y=0.5) -> (x+y=w427:dbl)
          }
        }
        n293 = case shown="True" w375 {
          tunnel: [w419 w422] -> w369
          tunnel: [w419 w421] -> w370
          tunnel: w373 -> [w419 w420]
          frame False {
          }
          frame True {
            n294 = Add(x=w420, y=230.0) -> (x+y=w422:dbl)
            n295 = Add(x=w420, y=0.5) -> (x+y=w421:dbl)
          }
        }
        n296 = case shown="True" w374 {
          tunnel: [w413 w416] -> w371
          tunnel: [w413 w415] -> w372
          tunnel: w373 -> [w413 w414]
          frame False {
          }
          frame True {
            n297 = Add(x=w414, y=230.0) -> (x+y=w416:dbl)
            n298 = Add(x=w414, y=0.5) -> (x+y=w415:dbl)
          }
        }
        n299 = case shown="True" w411 {
          tunnel: w373 -> [w479 w482]
          tunnel: [w479 w481] -> w408
          tunnel: [w479 w480] -> w407
          frame False {
          }
          frame True {
            n300 = Add(x=w482, y=230.0) -> (x+y=w480:dbl)
            n301 = Add(x=w482, y=1.5) -> (x+y=w481:dbl)
          }
        }
        n302 = case shown="True" w412 {
          tunnel: w373 -> [w485 w488]
          tunnel: [w485 w487] -> w410
          tunnel: [w485 w486] -> w409
          frame False {
          }
          frame True {
            n303 = Add(x=w488, y=230.0) -> (x+y=w487:dbl)
            n304 = Add(x=w488, y=0.5) -> (x+y=w486:dbl)
          }
        }
        n305 = case shown="True" w402 {
          tunnel: [w473 w476] -> w401
          tunnel: [w473 w475] -> w399
          tunnel: w373 -> [w473 w474]
          frame False {
          }
          frame True {
            n306 = Add(x=w474, y=230.0) -> (x+y=w476:dbl)
            n307 = Add(x=w474, y=0.5) -> (x+y=w475:dbl)
          }
        }
        n308 = case shown="True" w400 {
          tunnel: [w467 w470] -> w398
          tunnel: [w467 w469] -> w397
          tunnel: w373 -> [w467 w468]
          frame False {
          }
          frame True {
            n309 = Add(x=w468, y=230.0) -> (x+y=w470:dbl)
            n310 = Add(x=w468, y=0.5) -> (x+y=w469:dbl)
          }
        }
      }
    }
    "UL" <- w13
    "IL" <- w14
    n311 = local write "Thermometer\nConvertor"(w86) -> ()
    n312 = local read "Catlytic Valve"() -> (w78:bool)
    n313 = local read "COMPRESSOR"() -> (w81:dbl)
    n314 = local read "Catalityc Pump"() -> (w77:bool)
    n315 = Subtract(x=w132, y=w130) -> (x-y=w85:dbl)
    n316 = local read "OverPressure\nValve"() -> (w124:bool)
    n317 = Greater?(x=w81, y=1.0) -> (0:w79:bool)
    n318 = local write "Pressure2"(w124) -> ()
    n319 = Compound Arithmetic op=AND(w77, w78, w79) -> (w76:bool)
    n320 = case shown="True" w76 {
      selector: w76 -> [_ w249]
      tunnel: [0.0 0.001] -> w83
      tunnel: [FALSE w250] -> w82
      frame False {
      }
      frame True {
        n321 = case shown="True" w249 {
          tunnel: [FALSE TRUE] -> w250
          frame False {
          }
          frame True {
          }
        }
      }
    }
    n322 = Subtract(x=w85, y=w83) -> (x-y=w84:dbl)
    "ATM" <- w84
    n323 = Greater?(x=w84, y=2.0) -> (0:w125:bool)
    n324 = local write "Pressure1"(w125) -> ()
    n325 = local write "FINAL PRODUCT\nTANK"(w20) -> ()
    n326 = local write "RESIDUAL WATER \nTANK"(w19) -> ()
    n327 = local write "ABSORTION TOWER"(w55) -> ()
    n328 = local write "CATALYTIC \nCONVERTOR"(w66) -> ()
    n329 = local write "DILUTION TOWER"(w31) -> ()
    n330 = local write "U_av"(w99) -> ()
    n331 = local write "I_av"(w100) -> ()
    n332 = local write "U_ap"(w97) -> ()
    n333 = local write "Pressure"(w84) -> ()
    n334 = local write "U_ccv2"(w114) -> ()
    n335 = local write "I_ap"(w98) -> ()
    n336 = local write "U_ccv"(w110) -> ()
    n337 = local write "I_ccv"(w111) -> ()
    n338 = local write "U_ccp"(w112) -> ()
    n339 = local write "U_wp"(w118) -> ()
    n340 = local write "U_mp"(w121) -> ()
    n341 = local write "U_wv"(w116) -> ()
    n342 = local write "I_ccv2"(w115) -> ()
    n343 = local write "I_wp"(w119) -> ()
    n344 = local write "U_mv"(w123) -> ()
    n345 = local write "I_mp"(w120) -> ()
    n346 = local write "I_ccp"(w113) -> ()
    n347 = local write "I_wv"(w117) -> ()
    n348 = local write "I_mv"(w122) -> ()
    n349 = local write "Catalyst2"(w82) -> ()
    n350 = local write "U_sv"(w167) -> ()
    n351 = local write "U_opv"(w156) -> ()
    n352 = local write "U_cv"(w158) -> ()
    n353 = local write "U_sp"(w164) -> ()
    n354 = local write "I_opv"(w155) -> ()
    n355 = local write "I_sv"(w166) -> ()
    n356 = local write "I_cv"(w157) -> ()
    n357 = local write "I_sp"(w165) -> ()
    n358 = local write "IL"(w14) -> ()
    n359 = local write "UL"(w13) -> ()
    "Boolean" <- "SP"
    "Boolean 2" <- "SV"
    "Boolean 3" <- "FURN"
    "Boolean 4" <- "HV_SW"
    "Boolean 6" <- "CV"
    "Boolean 7" <- "OPV"
    "COMPRESSOR_ON" <- "COMP"
    "Boolean 5" <- "COMP"
    "Boolean 10" <- "CCV 2"
    "Boolean 12" <- "WV"
    "Boolean 11" <- "WP"
    "Boolean 13" <- "MP"
    "Boolean 8" <- "CCP"
    "Boolean 15" <- "AP"
    "Boolean 14" <- "MV"
    "Boolean 16" <- "AV"
    "Boolean 9" <- "CCV"
    "Boolean 17" <- "CONV"
    "Boolean 18" <- "TRANSFORMER"
    "TRANS" <- "TRANSFORMER"
  }
